vi "Pcre2SubstringFromSubjectByName8 (bsa).vi"(8 "error in":errorcluster, 9 "Name":string, 10 "Subject":string, 11 "pMatchData":u64 format="%.0x") -> (0 "error out":errorcluster, 2 "Substring":string, 3 "pMatchData":u64 format="%.0x", 4 "AfterSubstring":string, 5 "BeforeSubstring":string)   [LabVIEW 2021, in "libpcre2-8.lvlib"]
uses:
  libpcre2-8.lvlib
  Pcre2ErrorNull.vi
  Pcre2FnkCallError.vi
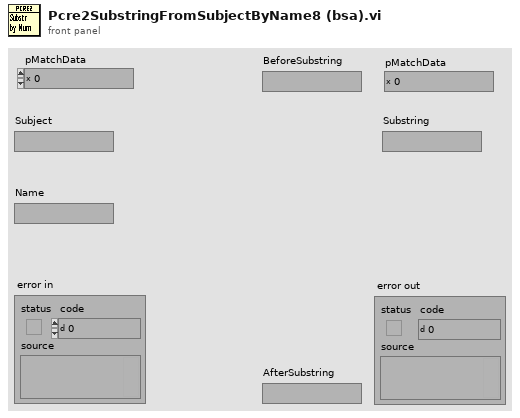
[diagram p1: front panel]
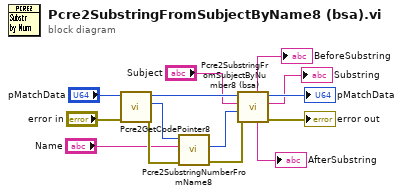
[diagram p0: block diagram]
diagram:
  n1 = call "Pcre2GetCodePointer8.vi"("error in"="error in", "pMatchData"="pMatchData") -> ("error out"=w13:errorcluster, "pCode"=w14:u64, "pMatchData"=w9:u64)  [unwired: 7 in]
  n2 = call "Pcre2SubstringNumberFromName8.vi"("error in"=w13, "Name"="Name", "pCode"=w14) -> ("error out"=w7:errorcluster, "Number"=w6:i32)  [unwired: 6 in, 1 out]
  n3 = call "Pcre2SubstringFromSubjectByNumber8 (bsa).vi"("error in"=w7, "Number"=w6, "Subject"="Subject", "pMatchData"=w9) -> ("error out"=→"error out":errorcluster, "Substring"=→"Substring":string, "pMatchData"=→"pMatchData":u64, "AfterSubstring"=→"AfterSubstring":string, "BeforeSubstring"=→"BeforeSubstring":string)  [unwired: 3 in]
